vi "Get 1D Subarray.vi"(1 "2D Array":dbl[][](array[numeric])=[[0.0, 9.0], [1.0, 8.0], [2.0, 7.0], [3.0, 6.0]] format="%0.8f", 3 "Row/Col":enum16{"Row", "Col"}(ring)=enum."Col", 5 "index":i32) -> (15 "1D Sub Array":dbl[](array[numeric]))   [LabVIEW 2014]
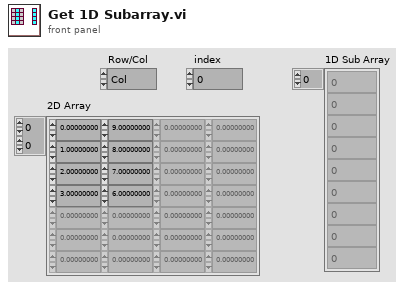
[diagram p1: front panel]
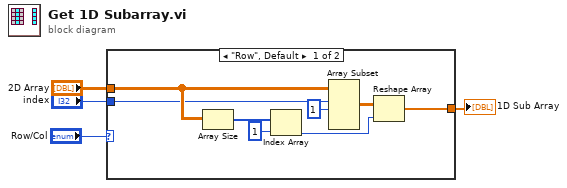
[diagram p0: block diagram]
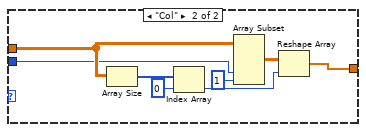
[diagram p2: hidden frame]
diagram:
  n1 = case shown="\"Row\", Default" "Row/Col" {
    tunnel: "2D Array" -> [w6 w20]
    tunnel: [w7 w15] -> w2
    tunnel: "index" -> [w5 w13]
    frame "Row", Default {
      n2 = Array Size(array=w6) -> (size(s)=w12:i32[])
      n3 = Index Array(array=w12, index=1) -> (element=w9:i32)
      n4 = Array Subset(array=w6, index (row)=w5, length (row)=1 ("length")) -> (w10:dbl[][])  [unwired: 2 in]
      n5 = Reshape Array(w10, w9) -> (w7:dbl[])
    }
    frame "Col" {
      n6 = Array Size(array=w20) -> (size(s)=w19:i32[])
      n7 = Index Array(array=w19, index=0) -> (element=w16:i32)
      n8 = Array Subset(array=w20, index (col)=w13, length (col)=1 ("length")) -> (w17:dbl[][])  [unwired: 2 in]
      n9 = Reshape Array(w17, w16) -> (w15:dbl[])
    }
  }
  "1D Sub Array" <- w2
